vi "Sets the Hi&Lo for MANU.vi"(0 "VISA resource name":refnum<visa-resource-name>, 1 "Number of MANU":i32=1 min=1 max=100 step=1, 2 "Enable to Setup":bool=TRUE, 3 "Enable to Query":bool, 5 "Hi Set Value":u32 step=1 format="%08x", 9 "Lo Set Value":u32 step=1 format="%08x", 11 "error in":errorcluster) -> (4 "VISA resource name out":refnum<visa-resource-name>, 6 "Return the Hi Value":u32 format="%08x", 10 "Return the Lo Value":u32 format="%08x", 15 "error out":errorcluster)   [LabVIEW 2011, in "GPT-9000.lvlib"]
uses:
  <instrlib>/GPT-9000/GPT-9000.lvlib
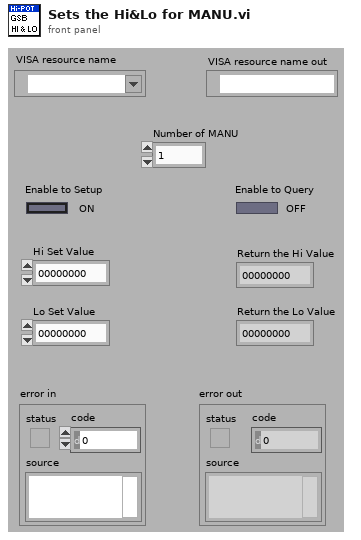
[diagram p1: front panel]
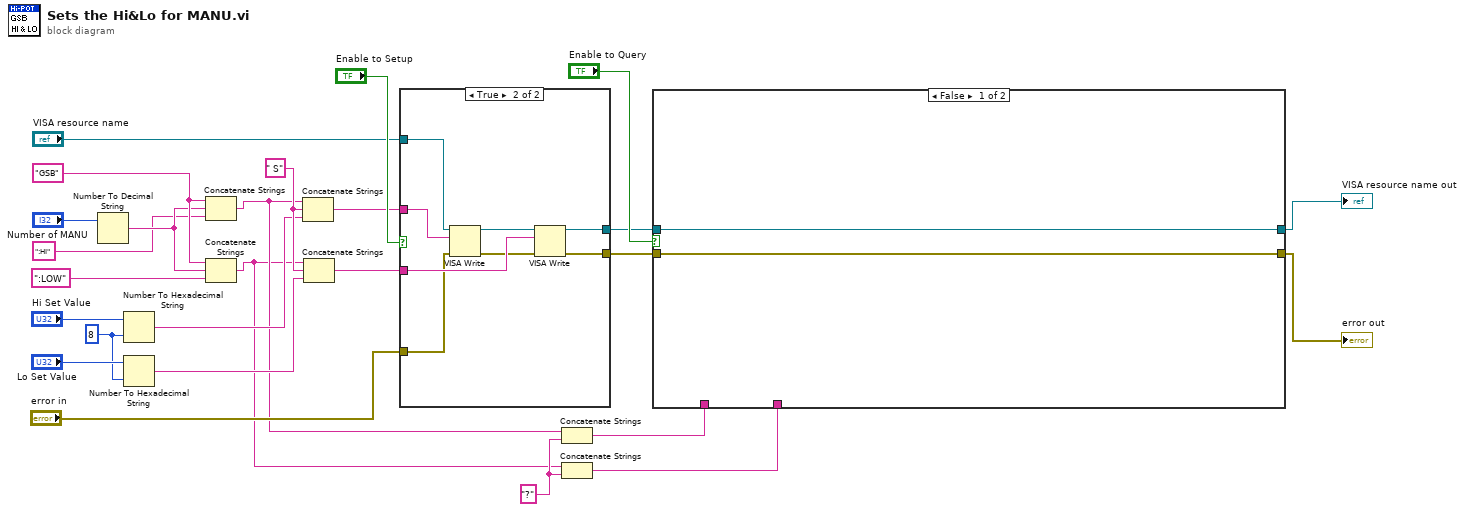
[diagram p0: block diagram]
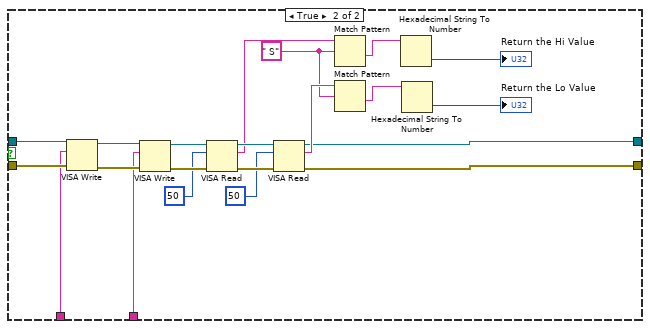
[diagram p2: hidden frame]
diagram:
  w1 = i16 8 ("width (-)")
  w11 = "?" ("string")
  w18 = " S" ("string")
  w24 = "GSB"
  n1 = Number To Decimal String(number="Number of MANU") -> (decimal integer string=w23:string)  [unwired: 1 in]
  n2 = Number To Hexadecimal String(1:w1, 2:"Hi Set Value") -> (0:w17:string)
  n3 = Number To Hexadecimal String(1:w1, 2:"Lo Set Value") -> (0:w16:string)
  n4 = Concatenate Strings(w24, w23, ":HI") -> (w10:string)
  n5 = Concatenate Strings(w24, w23, ":LOW") -> (w9:string)
  n6 = Concatenate Strings(w10, w18, w17) -> (w15:string)
  n7 = Concatenate Strings(w9, w18, w16) -> (w14:string)
  n8 = case shown="True" "Enable to Setup" {
    tunnel: w15 -> [_ w36]
    tunnel: w14 -> [_ w35]
    tunnel: "VISA resource name" -> [w28 w34]
    tunnel: "error in" -> [w27 w33]
    tunnel: [w28 w30] -> w7
    tunnel: [w27 w29] -> w6
    frame False {
    }
    frame True {
      n9 = VISA Write(VISA resource name=w34, write buffer=w36, error in (no error)=w33) -> (VISA resource name out=w32:refnum<visa-resource-name>, error out=w31:errorcluster)  [unwired: 1 out]
      n10 = VISA Write(VISA resource name=w32, write buffer=w35, error in (no error)=w31) -> (VISA resource name out=w30:refnum<visa-resource-name>, error out=w29:errorcluster)  [unwired: 1 out]
    }
  }
  n11 = Concatenate Strings(w10, w11) -> (w5:string)
  n12 = Concatenate Strings(w9, w11) -> (w4:string)
  n13 = case shown="False" "Enable to Query" {
    tunnel: w7 -> [w38 w59]
    tunnel: w6 -> [w37 w58]
    tunnel: w5 -> [_ w55]
    tunnel: w4 -> [_ w54]
    tunnel: [w38 w40] -> w3
    tunnel: [w37 w39] -> w2
    frame False {
    }
    frame True {
      w45 = " S"
      n14 = VISA Write(VISA resource name=w59, write buffer=w55, error in (no error)=w58) -> (VISA resource name out=w57:refnum<visa-resource-name>, error out=w56:errorcluster)  [unwired: 1 out]
      n15 = VISA Write(VISA resource name=w57, write buffer=w54, error in (no error)=w56) -> (VISA resource name out=w53:refnum<visa-resource-name>, error out=w51:errorcluster)  [unwired: 1 out]
      n16 = VISA Read(VISA resource name=w53, byte count=u32 50, error in (no error)=w51) -> (VISA resource name out=w52:refnum<visa-resource-name>, read buffer=w47:string, error out=w50:errorcluster)  [unwired: 1 out]
      n17 = VISA Read(VISA resource name=w52, byte count=u32 50, error in (no error)=w50) -> (VISA resource name out=w40:refnum<visa-resource-name>, read buffer=w46:string, error out=w39:errorcluster)  [unwired: 1 out]
      n18 = Match Pattern(string=w47, regular expression=w45) -> (after substring=w44:string)  [unwired: 1 in, 3 out]
      n19 = Match Pattern(string=w46, regular expression=w45) -> (after substring=w43:string)  [unwired: 1 in, 3 out]
      n20 = Hexadecimal String To Number(string=w44) -> (number=→"Return the Hi Value":u32)  [unwired: 2 in, 1 out]
      n21 = Hexadecimal String To Number(string=w43) -> (number=→"Return the Lo Value":u32)  [unwired: 2 in, 1 out]
    }
  }
  "VISA resource name out" <- w3
  "error out" <- w2
